vi "读取量程参数.vi"(8 "error in (no error)":errorcluster, 10 "引用选择":enum16{"MB引用", "自建引用"}(ring), 11 "MB session in":refnum<class "MB_Master.lvclass">) -> (0 "error out":errorcluster, 2 "自动测试量程配置":T2={"水样测试量程模式"=enum."H", "标样核查量程模式"=enum."H", "零点核查量程模式"=enum."H", "跨度核查量程模式"=enum."H", "空白测试量程模式"=enum."H", "平行样测试量程模式"=enum."H", "加标回收量程模式"=enum."H", "空白校准量程模式"=enum."H", "标样校准量程模式"=enum."H"}, 3 "MB session out":refnum<class "MB_Master.lvclass">)   [LabVIEW 2016, in "斯坦道CODMn新电路板.lvlib"]
uses:
  <vilib>/Plasmionique/MB Master/MB_Master/MB_Master.lvclass
  <vilib>/Plasmionique/MB Master/MB_Master_Serial/MB_Master_Serial.lvclass
  D:/Program Files (x86)/National Instruments/LabVIEW 2016/vi.lib/Plasmionique/MB Master/MB_Master/MB_Master.lvclass
  <vilib>/Plasmionique/MB Master/MB Master.lvlib
panel:
  in  "VISA Resource":refnum<visa-resource-name>
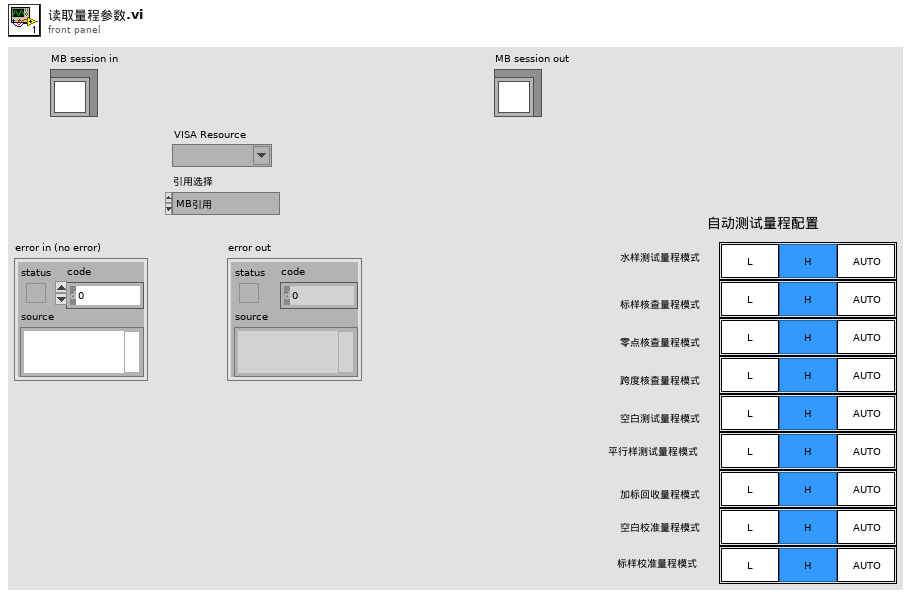
[diagram p1: front panel]
types:
  T1 = typedef "量程选择控件.ctl" = enum32{"L", "H", "AUTO"}
  T2 = cluster{"水样测试量程模式":T1, "标样核查量程模式":T1, "零点核查量程模式":T1, "跨度核查量程模式":T1, "空白测试量程模式":T1, "平行样测试量程模式":T1, "加标回收量程模式":T1, "空白校准量程模式":T1, "标样校准量程模式":T1}
  T3 = cluster{"baud rate (bps)":u32, "stop bits":u16, "parity":u16, "flow control":u16, "timeout":u32, "retries":i32}
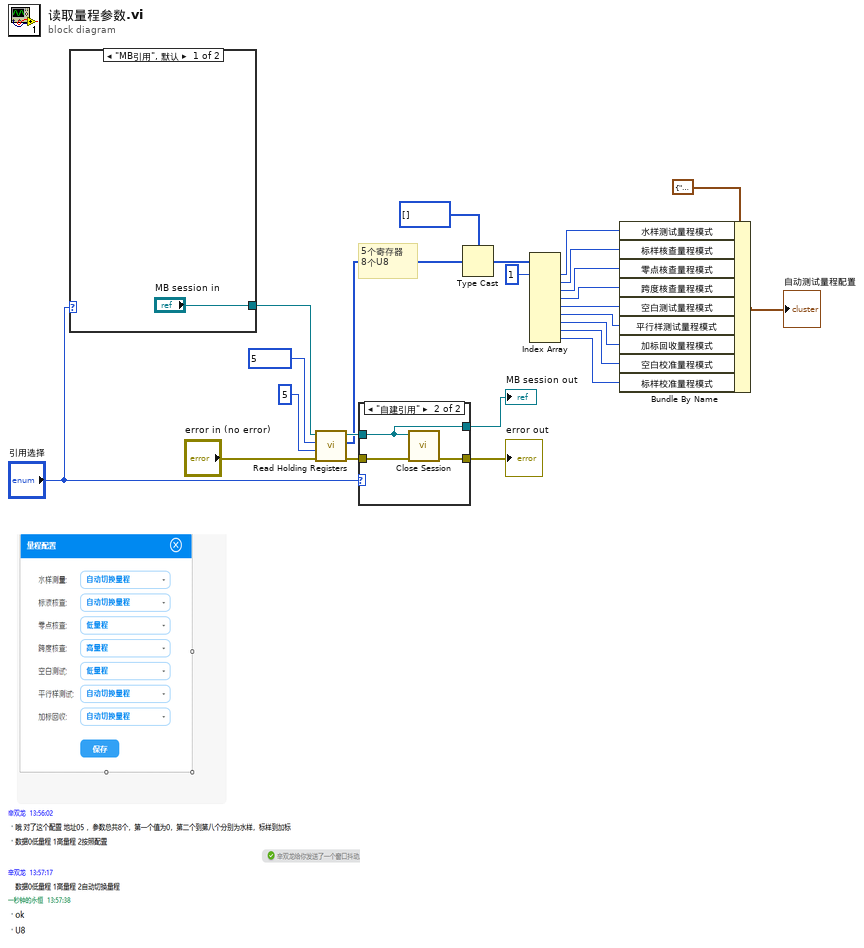
[diagram p0: block diagram]
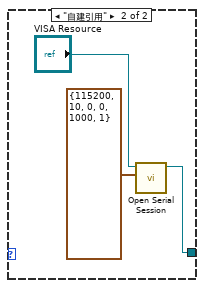
[diagram p3: hidden frame]
diagram:
  # "5个寄存器\n8个U8"
  n1 = case shown="\"MB引用\", 默认" "引用选择" {
    tunnel: ["MB session in" w28] -> w18
    frame "MB引用", Default {
    }
    frame "自建引用" {
      n2 = call <vilib>:"Open Serial Session.vi"("Serial Config"=T3 {"baud rate (bps)"=115200, "stop bits"=10, "parity"=0, "flow control"=0, "timeout"=1000, "retries"=1}, "VISA Resource"="VISA Resource") -> ("MB_Serial session"=w28:refnum<class "MB_Master_Serial.lvclass">)  [unwired: 8 in, 1 out]
    }
  }
  n3 = call <vilib>:"Read Holding Registers.vi"("error in (no error)"="error in (no error)", "quantity"=u16 5, "starting address"=u16 5, "MB session in"=w18) -> ("error out"=w15:errorcluster, "Registers"=w8:u16[], "MB session out"=w17:refnum<class "MB_Master.lvclass">)  [unwired: 5 in]
  n4 = case shown="\"自建引用\"" "引用选择" {
    tunnel: w17 -> [w29 w31]
    tunnel: w15 -> [w30 w33]
    tunnel: [w30 w32] -> w14
    tunnel: [w29 w31] -> w13
    frame "MB引用", Default {
    }
    frame "自建引用" {
      n5 = call-dynamic "Close Session.vi"("error in (no error)"=w33, "MB session in"=w31) -> ("error out"=w32:errorcluster)  [unwired: 9 in]
    }
  }
  "MB session out" <- w13
  "error out" <- w14
  n6 = Type Cast(type=u8[] [], x=w8) -> (*(type *) &x=w19:u8[])
  n7 = Index Array(array=w19, index #1=1 ("索引")) -> (element #1=w20:u8, element #2=w12:u8, element #3=w11:u8, element #4=w10:u8, element #5=w7:u8, element #6=w6:u8, element #7=w5:u8, element #8=w2:u8, element #9=w1:u8)  [unwired: 8 in]
  n8 = Bundle By Name(cluster=T2 {"水样测试量程模式"=enum."H", "标样核查量程模式"=enum."H", "零点核查量程模式"=enum."H", "跨度核查量程模式"=enum."H", "空白测试量程模式"=enum."H", "平行样测试量程模式"=enum."H", "加标回收量程模式"=enum."H", "空白校准量程模式"=enum."H", "标样校准量程模式"=enum."H"} ("自动测试量程配置"), "水样测试量程模式"=w20, "标样核查量程模式"=w12, "零点核查量程模式"=w11, "跨度核查量程模式"=w10, "空白测试量程模式"=w7, "平行样测试量程模式"=w6, "加标回收量程模式"=w5, "空白校准量程模式"=w2, "标样校准量程模式"=w1) -> (→"自动测试量程配置":T2)
